vi "Shoot Manual and Auto Management Vr2.vi"(0 "Auto Preparation for Shooting":bool, 1 "Le Fire At Will":bool, 5 "Pilot X":dbl, 7 "Pilot Y":dbl, 9 "Elevation":dbl, 11 "Shoot Motors":dbl, 12 "Stop Centerizing":bool, 13 "ReCenterize":bool, 14 "Fine Tune":bool) -> (6 "X Drive Arcade":dbl, 10 "Y Drive Arcade":dbl, 15 "Ready to Fire!":bool)   [LabVIEW 2012]
uses:
  Motors Values.vi
  BotStatus.vi
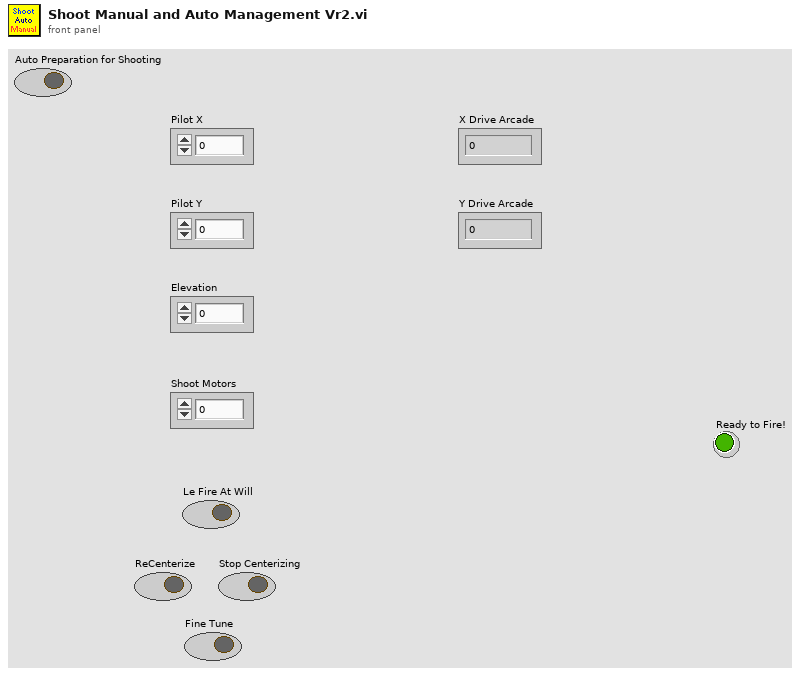
[diagram p1: front panel]
types:
  T1 = typedef "WPI_EncoderDevRef.ctl" = cluster{"DevStatus":errorcluster, "EncoderIndex":T2, "CounterIndex":T3, "DistancePerCount":dbl, "Decoding Type":T4}
  T2 = typedef "FPGA_EncoderIdx.ctl" = enum8{"Enc 0", "Enc 1", "Enc 2", "Enc 3", "Invalid"}
  T3 = typedef "FPGA_CounterCtrSystemIndex.ctl" = enum8{"Ctr 0", "Ctr 1", "Ctr 2", "Ctr 3", "Ctr 4", "Ctr 5", "Ctr 6", "Ctr 7", "Invalid"}
  T4 = typedef "WPI_EncoderType.ctl" = enum16{"1x", "2x", "4x"}
  T5 = cluster{"Middle":bool, "InCannon":bool, "InFlipper":bool, "FlipperAtPlace":bool, "Bottom":bool, "FrisbeeDirection":bool}
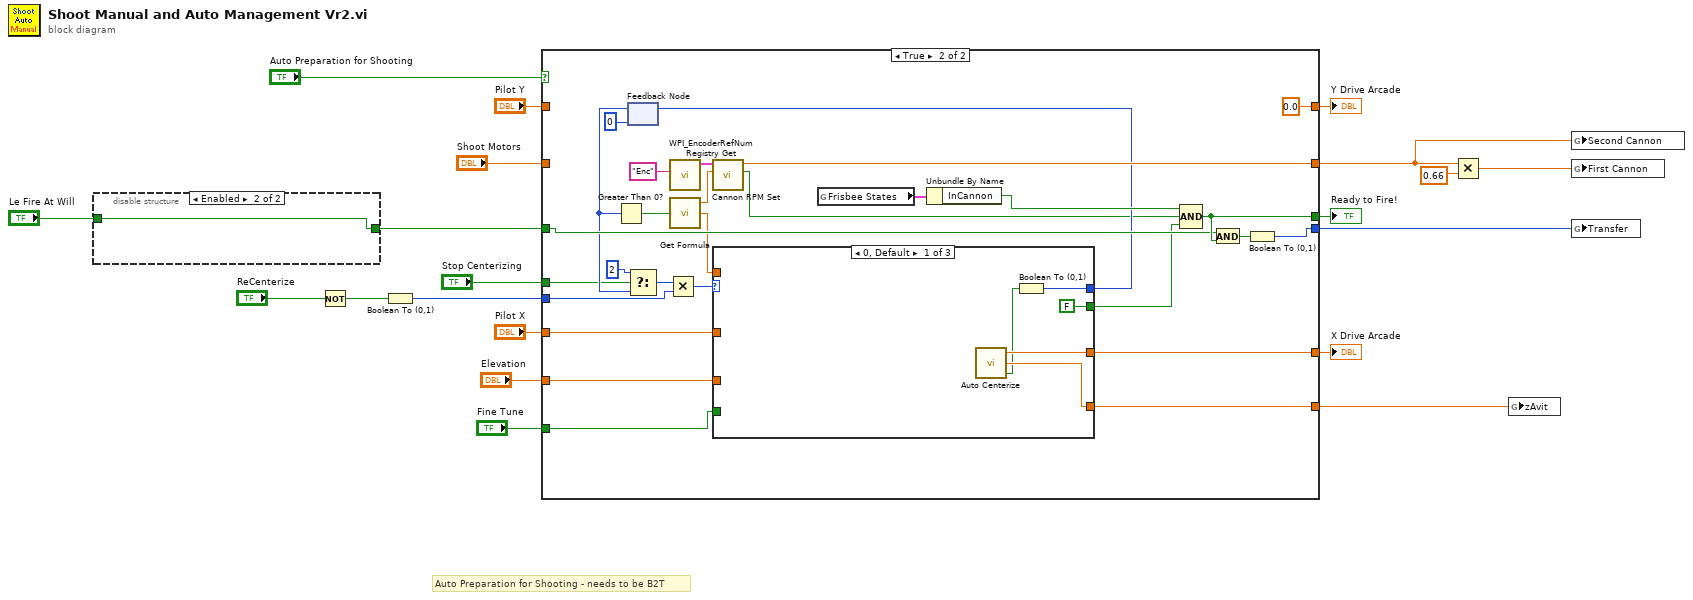
[diagram p0: block diagram]
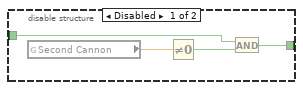
[diagram p2: hidden frame]
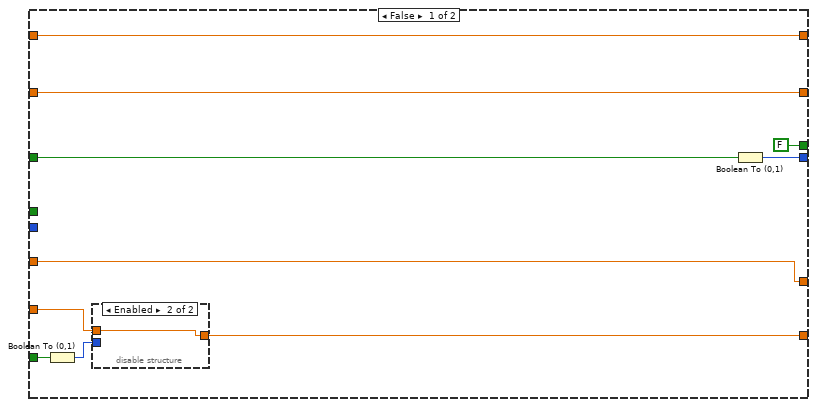
[diagram p3: hidden frame]
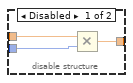
[diagram p4: hidden frame]
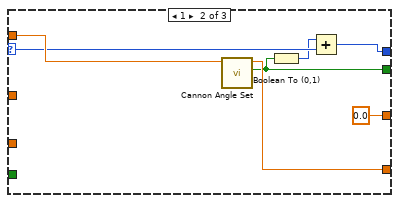
[diagram p5: hidden frame]
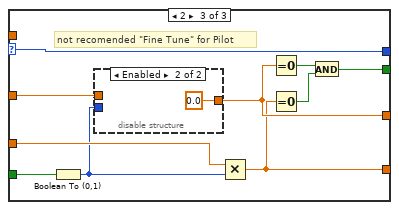
[diagram p6: hidden frame]
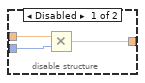
[diagram p7: hidden frame]
diagram:
  # "Auto Preparation for Shooting - needs to be B2T"
  n1 = disable-structure shown="Enabled" {
    disable-tunnel: "Le Fire At Will" -> [w22 w25]
    disable-tunnel: [w21 w25] -> w6
    frame Disabled {
      n2 = global read "Motors Values.vi" "Second Cannon"() -> (w24:dbl)
      n3 = Not Equal To 0?(x=w24) -> (x != 0?=w23:bool)
      n4 = And(x=w22, y=w23) -> (x .and. y?=w21:bool)
    }
    frame Enabled {
    }
  }
  n5 = Not(x="ReCenterize") -> (.not. x?=w2:bool)
  n6 = Boolean To (0,1)(Boolean=w2) -> (0, 1=w1:i16)
  n7 = case shown="True" "Auto Preparation for Shooting" {
    tunnel: [w30 w55] -> w17
    tunnel: [w35 w56] -> w18
    tunnel: "Pilot X" -> [w35 w48]
    tunnel: "Elevation" -> [w34 w49]
    tunnel: w6 -> [w28 w58]
    tunnel: [w33 w65] -> w15
    tunnel: [w32 w64] -> w12
    tunnel: "Shoot Motors" -> [w32 _]
    tunnel: "Pilot Y" -> [w31 _]
    tunnel: [w31 0.0] -> w9
    tunnel: [FALSE w59] -> w8
    tunnel: "Fine Tune" -> [w26 w50]
    tunnel: "Stop Centerizing" -> [_ w46]
    tunnel: w1 -> [_ w42]
    frame False {
      n8 = Boolean To (0,1)(Boolean=w26) -> (0, 1=w29:i16)
      n9 = disable-structure shown="Enabled" {
        disable-tunnel: w34 -> [w38 w39]
        disable-tunnel: [w37 w39] -> w30
        disable-tunnel: w29 -> [w36 _]
        frame Disabled {
          n10 = Multiply(x=w38, y=w36) -> (x*y=w37:dbl)
        }
        frame Enabled {
        }
      }
      n11 = Boolean To (0,1)(Boolean=w28) -> (0, 1=w33:i16)
    }
    frame True {
      n12 = feedback #1(0) -> (w47:i32)
      n13 = Greater Than 0?(x=w47) -> (x > 0?=w51:bool)
      n14 = Select(t=2, s=w46, f=w47) -> (s? t:f=w43:i32)
      n15 = Multiply(x=w43, y=w42) -> (x*y=w44:i32)
      n16 = call <vilib>:"WPI_EncoderRefNum Registry Get.vi"("refnum name"="Enc") -> ("EncoderDevRef"=w61:T1)  [unwired: 9 in, 1 out]
      n17 = call "Get Formula.vi"("Make Formula"=w51) -> ("Cannon Angle Set Point"=w52:dbl, "RPM Set Point"=w53:dbl)  [unwired: 2 in, 1 out]
      n18 = call "Cannon RPM Set.vi"("Set Point RPM"=w53, "EncoderDevRef"=w61) -> ("READY!"=w41:bool, "Vbus Out"=w64:dbl)  [unwired: 8 in]
      n19 = case shown="0, Default" w44 {
        selector: w44 -> [_ w76 w85]
        tunnel: [w72 0.0 ("X Drive Arcade") w84] -> w56
        tunnel: [w71 w78 w83] -> w55
        tunnel: [w69 w74 w85] -> w54
        tunnel: w52 -> [_ w79 _]
        tunnel: w50 -> [_ _ w89]
        tunnel: w49 -> [_ _ w88]
        tunnel: w48 -> [_ _ w87]
        tunnel: [FALSE ("On Target") w73 w80] -> w40
        frame 0, Default {
          n20 = call "Auto Centerize.vi"() -> ("Centerized?"=w70:bool, "zAvit"=w71:dbl, "X Drive Arcade"=w72:dbl)  [unwired: 3 in]
          n21 = Boolean To (0,1)(Boolean=w70) -> (0, 1=w69:i16)
        }
        frame 1 {
          n22 = call "Cannon Angle Set.vi"("Angle Set Point"=w79) -> ("On Target"=w73:bool, "zAvit Vbus Out"=w78:dbl)  [unwired: 9 in]
          n23 = Boolean To (0,1)(Boolean=w73) -> (0, 1=w75:i16)
          n24 = Add(x=w75, y=w76) -> (x+y=w74:i32)
        }
        frame 2 {
          # "not recomended \"Fine Tune\" for Pilot"
          n25 = Boolean To (0,1)(Boolean=w89) -> (0, 1=w86:i16)
          n26 = disable-structure shown="Enabled" {
            disable-tunnel: w87 -> [w92 _]
            disable-tunnel: w86 -> [w91 _]
            disable-tunnel: [w90 0.0] -> w84
            frame Disabled {
              n27 = Multiply(x=w92, y=w91) -> (x*y=w90:dbl)
            }
            frame Enabled {
            }
          }
          n28 = Multiply(x=w88, y=w86) -> (x*y=w83:dbl)
          n29 = Equal To 0?(x=w84) -> (x = 0?=w81:bool)
          n30 = Equal To 0?(x=w83) -> (x = 0?=w82:bool)
          n31 = And(x=w81, y=w82) -> (x .and. y?=w80:bool)
        }
      }
      n32 = feedback-in #1(w54) -> ()
      n33 = global read "BotStatus.vi" "Frisbee States"() -> (w67:T5)
      n34 = Unbundle By Name(w67) -> ("InCannon"=w66:bool)
      n35 = Compound Arithmetic op=AND(w66, w41, w40) -> (w59:bool)
      n36 = And(x=w58, y=w59) -> (x .and. y?=w60:bool)
      n37 = Boolean To (0,1)(Boolean=w60) -> (0, 1=w65:i16)
    }
  }
  "X Drive Arcade" <- w18
  "Y Drive Arcade" <- w9
  "Ready to Fire!" <- w8
  n38 = Multiply(x=w12, y=0.66) -> (x*y=w13:dbl)
  n39 = global write "Motors Values.vi" "zAvit"(w17) -> ()
  n40 = global write "Motors Values.vi" "Second Cannon"(w12) -> ()
  n41 = global write "Motors Values.vi" "First Cannon"(w13) -> ()
  n42 = global write "Motors Values.vi" "Transfer"(w15) -> ()
